vi "Split and Invert u16 to two u8.vi"(8 "Invert LSB [F]":bool, 9 "Invert MSB [F]":bool, 10 "Input (u16)":u16) -> (0 "Output(u16)":u32, 1 "LSB (u8)":u8, 2 "MSB (u8)":u8)   [LabVIEW 2025]
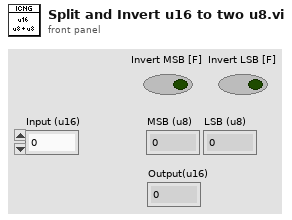
[diagram p1: front panel]
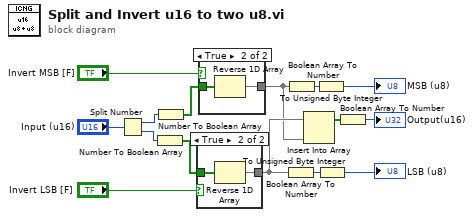
[diagram p0: block diagram]
diagram:
  n1 = Split Number(x="Input (u16)") -> (hi(x)=w13:u8, lo(x)=w12:u8)
  n2 = Number To Boolean Array(number=w12) -> (Boolean array=w15:bool[])
  n3 = Number To Boolean Array(number=w13) -> (Boolean array=w14:bool[])
  n4 = case shown="True" "Invert LSB [F]" {
    tunnel: w15 -> [w16 w18]
    tunnel: [w16 w17] -> w2
    frame False {
    }
    frame True {
      n5 = Reverse 1D Array(array=w18) -> (reversed array=w17:bool[])
    }
  }
  n6 = case shown="True" "Invert MSB [F]" {
    tunnel: w14 -> [w19 w21]
    tunnel: [w19 w20] -> w1
    frame False {
    }
    frame True {
      n7 = Reverse 1D Array(array=w21) -> (reversed array=w20:bool[])
    }
  }
  n8 = Boolean Array To Number(Boolean array=w2) -> (number=w9:u32)
  n9 = Boolean Array To Number(Boolean array=w1) -> (number=w10:u32)
  n10 = Insert Into Array(array=w2, new element=w1) -> (w4:bool[])  [unwired: 1 in]
  n11 = To Unsigned Byte Integer(number=w10) -> (unsigned 8bit integer=→"MSB (u8)":u8)
  n12 = To Unsigned Byte Integer(number=w9) -> (unsigned 8bit integer=→"LSB (u8)":u8)
  n13 = Boolean Array To Number(Boolean array=w4) -> (number=→"Output(u16)":u32)
